vi "AuMT8852B Carrier Drift Test Configuration.vi"(5 "Settings":T1={"Low frequency selection"=enum."Use low frequency", "Medium frequency selection"=enum."Don't use medium frequency", "High frequency selection"=enum."Don't use high frequency", "Low TX frequency"=2402.0, "Medium TX frequency"=2441.0, "High TX frequency"=2480.0, "Number of packets"=10, "Hop selection"=enum."Test with hopping on", "DH1 selection"=enum."Test with DH1 packets", "DH3 selection"=enum."Test with DH3 packets", "DH5 selection"=enum."Test with DH5 packets", "1-slot packet drift limit"=25000.0, "3-slot packet drift limit"=40000.0, "5-slot packet drift limit"=40000.0, "Drift rate limit"=20000.0, "Test control"=enum."Loopback", "Hop mode"=enum."Defined", "Null packet drift limit"=20000.0, "Low RX frequency"=2480.0, "Medium RX frequency"=2402.0, "High RX frequency"=2402.0}, 7 "Set/Get (Set)":enum16{"Set", "Get"}(ring), 8 "error in (no error)":errorcluster, 10 "Script (3)":i32=3, 11 "VISA session":refnum<visa-resource-name>) -> (0 "error out":errorcluster, 2 "error code":i32, 3 "VISA session out":refnum<visa-resource-name>, 4 "Settings out":T1={"Low frequency selection"=enum."Use low frequency", "Medium frequency selection"=enum."Use medium frequency", "High frequency selection"=enum."Use high frequency", "Low TX frequency"=0.0, "Medium TX frequency"=0.0, "High TX frequency"=0.0, "Number of packets"=0, "Hop selection"=enum."Test with hopping on", "DH1 selection"=enum."Test with DH1 packets", "DH3 selection"=enum."Test with DH3 packets", "DH5 selection"=enum."Test with DH5 packets", "1-slot packet drift limit"=0.0, "3-slot packet drift limit"=0.0, "5-slot packet drift limit"=0.0, "Drift rate limit"=0.0, "Test control"=enum."Loopback", "Hop mode"=enum."Any", "Null packet drift limit"=0.0, "Low RX frequency"=0.0, "Medium RX frequency"=0.0, "High RX frequency"=0.0})   [LabVIEW 2017]
doc: "Anritsu MT8852B Bluetooth Tester\n\nConfigures the instrument for the Carrier Drift test.\n\nINPUTS\nSet/Get - whether the values are being sent to or retrieved from the instrument.\nScript - which of the stored scripts (1-10) will be queried or configured. Scripts 1 and 2 are read-only.\nSettings - parameters of the test to be written.\n\nOUTPUTS\nSettings out - current parameters of the test."
uses:
  <instrlib>/aumt8852B/General/Utilities/MT8850 Test Parameters.ctl
  <instrlib>/aumt8852B/General/Utilities/MT8850 Frequency Units.ctl
panel:
  in  "Case Constant\n(See Context Help)":bool
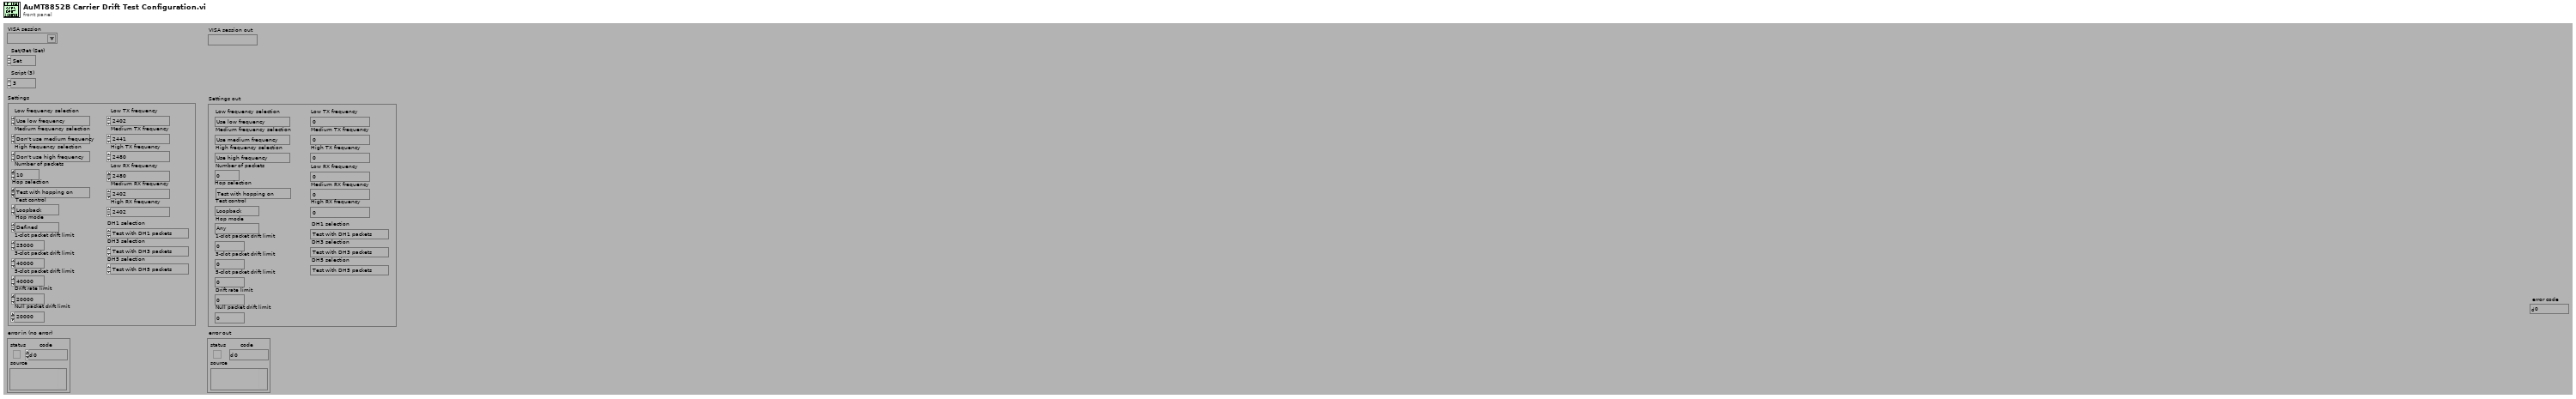
[diagram p1: front panel]
types:
  T1 = cluster{"Low frequency selection":enum16{"Don't use low frequency", "Use low frequency"}, "Medium frequency selection":enum16{"Don't use medium frequency", "Use medium frequency"}, "High frequency selection":enum16{"Don't use high frequency", "Use high frequency"}, "Low TX frequency":dbl, "Medium TX frequency":dbl, "High TX frequency":dbl, "Number of packets":i32, "Hop selection":enum16{"Test with hopping on", "Test with hopping off", "Test with hopping on and off"}, "DH1 selection":enum16{"Don't test with DH1 packets", "Test with DH1 packets"}, "DH3 selection":enum16{"Don't test with DH3 packets", "Test with DH3 packets"}, "DH5 selection":enum16{"Don't test with DH5 packets", "Test with DH5 packets"}, "1-slot packet drift limit":dbl, "3-slot packet drift limit":dbl, "5-slot packet drift limit":dbl, "Drift rate limit":dbl, "Test control":enum16{"Loopback", "TX test"}, "Hop mode":enum16{"All", "Any", "Defined"}, "Null packet drift limit":dbl, "Low RX frequency":dbl, "Medium RX frequency":dbl, "High RX frequency":dbl}
  T2 = typedef "MT8850 Test Parameters.ctl" = enum16{"Use low frequency", "Use medium frequency", "Use high frequency", "Low TX frequency", "Low RX frquency", "Medium TX frequency", "Medium RX frequency", "High TX frequency", "High RX frequency", "Number of packets", "Average high limit", "Average low limit", "Peak power limit", "Max power step limit", "Min power step limit", "f1 average minimum", "f1 average maximum", "f2 maximum", "f1/f2 average maximum", "Hop selection", "Use DH1 packets", "Use DH3 packets", "Use DH5 packets", "1 slot packet drift limit", "3 slot packet drift limit", "5 slot packet drift limit", "Drift rate limit", "TX power level", "Frequency offset", "Symbol timing", "Modulation index", "BER limit", "FER limit", "Use averaging high limit", "Use averaging low limit", "Use peak power limit", "Packet type", "Test control", "Use max power step limit", "Use min power step limit", "Number of cycles", "Use f1 average maximum", "Use f1 average minimum", "Use f2 maximum", "Use f1/f2 average maximum", "Hop mode", "Maximum negative limit", "Maximum positive limit", "Use maximum negative limit", "Use maximum positive limit", "Use 1 slot packet drift limit", "Use 3 slot packet drift limit", "Use 5 slot packet drift limit", "Use drift rate limit", "Use BER limit", "Use FER limit", "Use dirty parameter table", "Use null packet drift limit", "Null packet drift limit", "Minimum power", "Power delay", "Packet count", "Payload toggle", "Output power level", "2DHX packet type", "3DHX packet type", "Number of blocks", "TX and RX low frequency", "TX and RX medium frequency", "TX and RX high frequency", "TX frequency", "RX frequency", "Threshold bit count", "Total test bit count", "Number of bits", "PDPSK to PGFSK lower limit", "PDPSK to PGFSK upper limit", "Initial frequency error upper limit", "Initial frequency error lower limit", "Frequency error upper limit", "Frequency error lower limit", "Block frequency error upper limit", "Block frequency error lower limit", "2Mbs RMS DEVM limit", "3Mbs RMS DEVM limit", "2Mbs Peak DEVM limit", "3Mbs Peak DEVM limit", "2Mbs 99% packets DEVM limit", "3Mbs 99% packets DEVM limit", "Percentage of no error packets limit", "Threshold error limit", "Total test error limit"}
  T3 = typedef "MT8850 Frequency Units.ctl" = enum16{"Channel", "Hz", "kHz", "MHz", "GHz"}
  T4 = enum16{"Simulate", "Range check", "Cache", "Query instrument status"}
  T5 = enum16{"Output power", "Power control", "Modulation characteristics", "Initial carrier", "Carrier drift", "Single slot sensitivity", "Multiple slot sensitivity", "Maximum input power"}
  T6 = enum16{"Don't test with DH5 packets", "Test with DH5 packets"}
  T7 = enum16{"Don't test with DH3 packets", "Test with DH3 packets"}
  T8 = enum16{"Don't test with DH1 packets", "Test with DH1 packets"}
  T9 = enum16{"Test with hopping on", "Test with hopping off", "Test with hopping on and off"}
  T10 = enum16{"Don't use high frequency", "Use high frequency"}
  T11 = enum16{"Don't use medium frequency", "Use medium frequency"}
  T12 = enum16{"Don't use low frequency", "Use low frequency"}
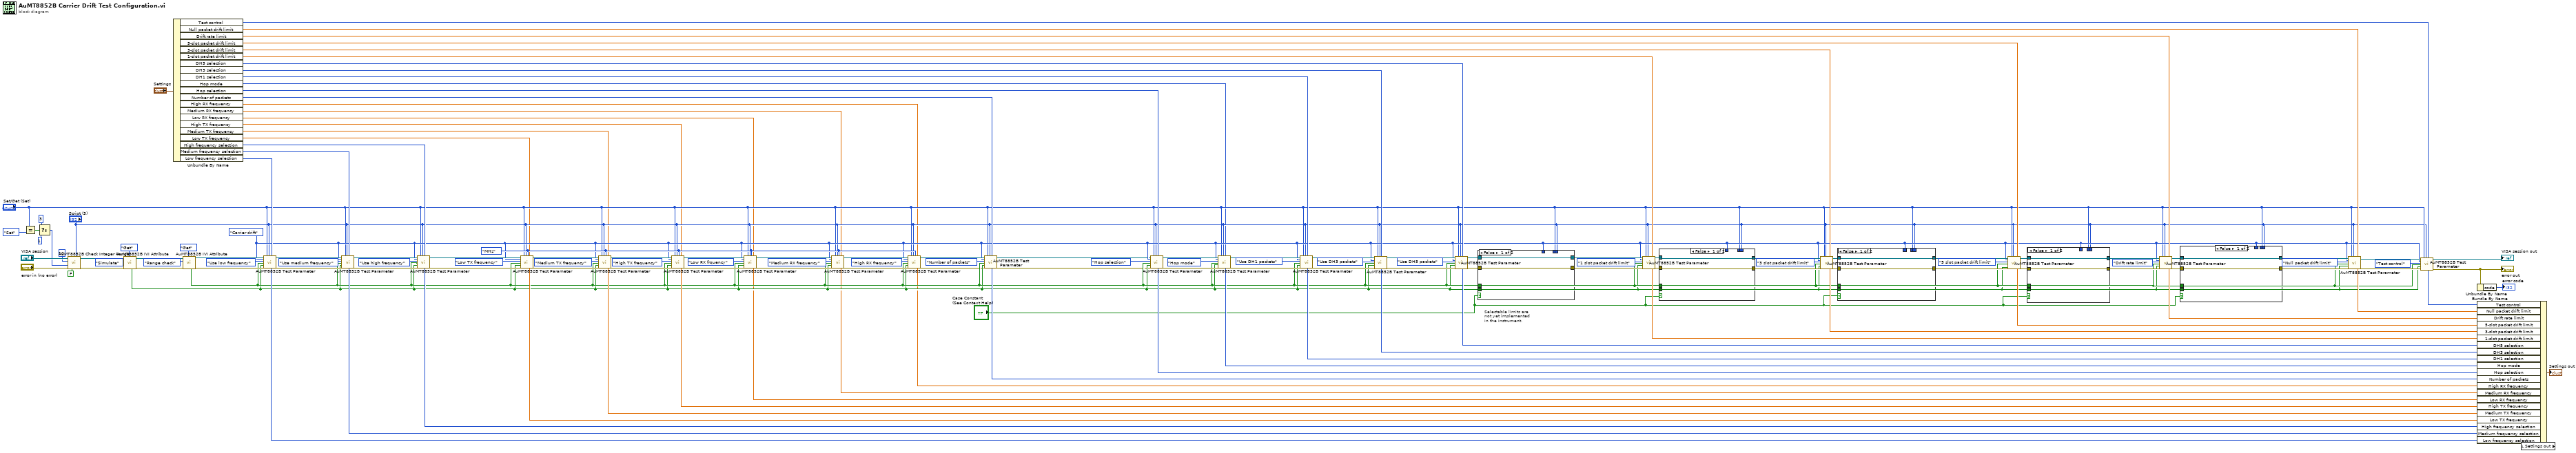
[diagram p0: block diagram]
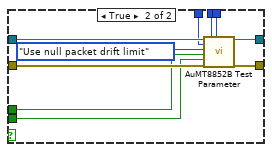
[diagram p2: hidden frame]
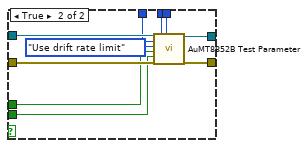
[diagram p3: hidden frame]
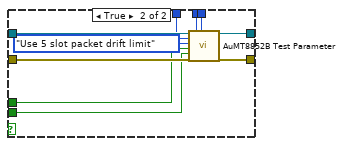
[diagram p4: hidden frame]
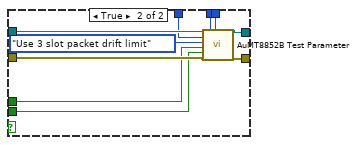
[diagram p5: hidden frame]
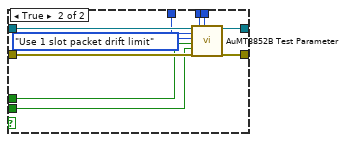
[diagram p6: hidden frame]
diagram:
  w20 = MT8850_Frequency_Units."MHz" ("Frequency units (MHz)")
  w15 = T5."Carrier drift" ("Test (Output Power)")
  # "Selectable limits are\nnot yet implemented\nin the instrument."
  n1 = Equal?(x="Set/Get (Set)", y=enum16{"Set", "Get"}."Set") -> (x = y?=w142:bool)
  n2 = Select(t=3, s=w142, f=1) -> (s? t:f=w138:i32)
  n3 = call <instrlib>:"AuMT8852B Check Integer Range.vi"("Value (0)"="Script (3)", "Check IVI flag first? (T)"=FALSE, "error in (no error)"="error in (no error)", "Lower limit (-1)"=w138, "Upper limit (1)"=10, "VISA session"="VISA session") -> ("error out"=w136:errorcluster, "VISA session out"=w137:refnum<visa-resource-name>)  [unwired: 4 in]
  n4 = call <instrlib>:"AuMT8852B IVI Attribute.vi"("Set/Get (Set)"=enum16{"Set", "Get"}."Get", "error in (no error)"=w136, "Flag (Simulate)"=T4."Simulate", "VISA session"=w137) -> ("error out"=w117:errorcluster, "VISA session out"=w118:refnum<visa-resource-name>, "Value out"=w18:bool)  [unwired: 5 in]
  n5 = Unbundle By Name("Settings") -> ("Test control"=w33:enum16{"Loopback", "TX test"}, "Null packet drift limit"=w34:dbl, "Drift rate limit"=w83:dbl, "5-slot packet drift limit"=w84:dbl, "3-slot packet drift limit"=w85:dbl, "1-slot packet drift limit"=w86:dbl, "DH5 selection"=w87:T6, "DH3 selection"=w88:T7, "DH1 selection"=w89:T8, "Hop mode"=w1:enum16{"All", "Any", "Defined"}, "Hop selection"=w96:T9, "Number of packets"=w108:i32, "High RX frequency"=w9:dbl, "Medium RX frequency"=w8:dbl, "Low RX frequency"=w2:dbl, "High TX frequency"=w10:dbl, "Medium TX frequency"=w11:dbl, "Low TX frequency"=w12:dbl, "High frequency selection"=w109:T10, "Medium frequency selection"=w110:T11, "Low frequency selection"=w111:T12)
  n6 = call <instrlib>:"AuMT8852B IVI Attribute.vi"("Set/Get (Set)"=enum16{"Set", "Get"}."Get", "error in (no error)"=w117, "Flag (Simulate)"=T4."Range check", "VISA session"=w118) -> ("error out"=w115:errorcluster, "VISA session out"=w116:refnum<visa-resource-name>, "Value out"=w19:bool)  [unwired: 5 in]
  n7 = call <instrlib>:"AuMT8852B Test Parameter.vi"("VISA session"=w116, "Test (Output power)"=w15, "Parameter (Use low frequency)"=MT8850_Test_Parameters."Use low frequency", "Range check? (F)"=w19, "Simulate? (F)"=w18, "error in (no error)"=w115, "Set/Get (Set)"="Set/Get (Set)", "Script (3)"="Script (3)", "Integer value (0)"=w111) -> ("Integer value out"=w100:i32, "VISA session out"=w49:refnum<visa-resource-name>, "error out"=w48:errorcluster)  [unwired: 7 in, 1 out]
  n8 = call <instrlib>:"AuMT8852B Test Parameter.vi"("VISA session"=w49, "Test (Output power)"=w15, "Parameter (Use low frequency)"=MT8850_Test_Parameters."Use medium frequency", "Range check? (F)"=w19, "Simulate? (F)"=w18, "error in (no error)"=w48, "Set/Get (Set)"="Set/Get (Set)", "Script (3)"="Script (3)", "Integer value (0)"=w110) -> ("Integer value out"=w101:i32, "VISA session out"=w47:refnum<visa-resource-name>, "error out"=w46:errorcluster)  [unwired: 7 in, 1 out]
  n9 = call <instrlib>:"AuMT8852B Test Parameter.vi"("VISA session"=w47, "Test (Output power)"=w15, "Parameter (Use low frequency)"=MT8850_Test_Parameters."Use high frequency", "Range check? (F)"=w19, "Simulate? (F)"=w18, "error in (no error)"=w46, "Set/Get (Set)"="Set/Get (Set)", "Script (3)"="Script (3)", "Integer value (0)"=w109) -> ("Integer value out"=w102:i32, "VISA session out"=w132:refnum<visa-resource-name>, "error out"=w131:errorcluster)  [unwired: 7 in, 1 out]
  n10 = call <instrlib>:"AuMT8852B Test Parameter.vi"("VISA session"=w132, "Test (Output power)"=w15, "Parameter (Use low frequency)"=MT8850_Test_Parameters."Low TX frequency", "Range check? (F)"=w19, "Simulate? (F)"=w18, "error in (no error)"=w131, "Set/Get (Set)"="Set/Get (Set)", "Script (3)"="Script (3)", "Integer value (0)"=w20, "Float value (0)"=w12) -> ("Float value out"=w103:dbl, "VISA session out"=w130:refnum<visa-resource-name>, "error out"=w129:errorcluster)  [unwired: 6 in, 1 out]
  n11 = call <instrlib>:"AuMT8852B Test Parameter.vi"("VISA session"=w130, "Test (Output power)"=w15, "Parameter (Use low frequency)"=MT8850_Test_Parameters."Medium TX frequency", "Range check? (F)"=w19, "Simulate? (F)"=w18, "error in (no error)"=w129, "Set/Get (Set)"="Set/Get (Set)", "Script (3)"="Script (3)", "Integer value (0)"=w20, "Float value (0)"=w11) -> ("Float value out"=w104:dbl, "VISA session out"=w128:refnum<visa-resource-name>, "error out"=w127:errorcluster)  [unwired: 6 in, 1 out]
  n12 = call <instrlib>:"AuMT8852B Test Parameter.vi"("VISA session"=w128, "Test (Output power)"=w15, "Parameter (Use low frequency)"=MT8850_Test_Parameters."High TX frequency", "Range check? (F)"=w19, "Simulate? (F)"=w18, "error in (no error)"=w127, "Set/Get (Set)"="Set/Get (Set)", "Script (3)"="Script (3)", "Integer value (0)"=w20, "Float value (0)"=w10) -> ("Float value out"=w105:dbl, "VISA session out"=w22:refnum<visa-resource-name>, "error out"=w21:errorcluster)  [unwired: 6 in, 1 out]
  n13 = call <instrlib>:"AuMT8852B Test Parameter.vi"("VISA session"=w22, "Test (Output power)"=w15, "Parameter (Use low frequency)"=MT8850_Test_Parameters."Low RX frquency", "Range check? (F)"=w19, "Simulate? (F)"=w18, "error in (no error)"=w21, "Set/Get (Set)"="Set/Get (Set)", "Script (3)"="Script (3)", "Integer value (0)"=w20, "Float value (0)"=w2) -> ("Float value out"=w5:dbl, "VISA session out"=w23:refnum<visa-resource-name>, "error out"=w24:errorcluster)  [unwired: 6 in, 1 out]
  n14 = call <instrlib>:"AuMT8852B Test Parameter.vi"("VISA session"=w23, "Test (Output power)"=w15, "Parameter (Use low frequency)"=MT8850_Test_Parameters."Medium RX frequency", "Range check? (F)"=w19, "Simulate? (F)"=w18, "error in (no error)"=w24, "Set/Get (Set)"="Set/Get (Set)", "Script (3)"="Script (3)", "Integer value (0)"=w20, "Float value (0)"=w8) -> ("Float value out"=w6:dbl, "VISA session out"=w25:refnum<visa-resource-name>, "error out"=w26:errorcluster)  [unwired: 6 in, 1 out]
  n15 = call <instrlib>:"AuMT8852B Test Parameter.vi"("VISA session"=w25, "Test (Output power)"=w15, "Parameter (Use low frequency)"=MT8850_Test_Parameters."High RX frequency", "Range check? (F)"=w19, "Simulate? (F)"=w18, "error in (no error)"=w26, "Set/Get (Set)"="Set/Get (Set)", "Script (3)"="Script (3)", "Integer value (0)"=w20, "Float value (0)"=w9) -> ("Float value out"=w7:dbl, "VISA session out"=w16:refnum<visa-resource-name>, "error out"=w17:errorcluster)  [unwired: 6 in, 1 out]
  n16 = call <instrlib>:"AuMT8852B Test Parameter.vi"("VISA session"=w16, "Test (Output power)"=w15, "Parameter (Use low frequency)"=MT8850_Test_Parameters."Number of packets", "Range check? (F)"=w19, "Simulate? (F)"=w18, "error in (no error)"=w17, "Set/Get (Set)"="Set/Get (Set)", "Script (3)"="Script (3)", "Integer value (0)"=w108) -> ("Integer value out"=w106:i32, "VISA session out"=w4:refnum<visa-resource-name>, "error out"=w3:errorcluster)  [unwired: 7 in, 1 out]
  n17 = call <instrlib>:"AuMT8852B Test Parameter.vi"("VISA session"=w4, "Test (Output power)"=w15, "Parameter (Use low frequency)"=MT8850_Test_Parameters."Hop selection", "Range check? (F)"=w19, "Simulate? (F)"=w18, "error in (no error)"=w3, "Set/Get (Set)"="Set/Get (Set)", "Script (3)"="Script (3)", "Integer value (0)"=w96) -> ("Integer value out"=w95:i32, "VISA session out"=w126:refnum<visa-resource-name>, "error out"=w125:errorcluster)  [unwired: 7 in, 1 out]
  n18 = call <instrlib>:"AuMT8852B Test Parameter.vi"("VISA session"=w126, "Test (Output power)"=w15, "Parameter (Use low frequency)"=MT8850_Test_Parameters."Hop mode", "Range check? (F)"=w19, "Simulate? (F)"=w18, "error in (no error)"=w125, "Set/Get (Set)"="Set/Get (Set)", "Script (3)"="Script (3)", "Integer value (0)"=w1) -> ("Integer value out"=w94:i32, "VISA session out"=w99:refnum<visa-resource-name>, "error out"=w98:errorcluster)  [unwired: 7 in, 1 out]
  n19 = call <instrlib>:"AuMT8852B Test Parameter.vi"("VISA session"=w99, "Test (Output power)"=w15, "Parameter (Use low frequency)"=MT8850_Test_Parameters."Use DH1 packets", "Range check? (F)"=w19, "Simulate? (F)"=w18, "error in (no error)"=w98, "Set/Get (Set)"="Set/Get (Set)", "Script (3)"="Script (3)", "Integer value (0)"=w89) -> ("Integer value out"=w70:i32, "VISA session out"=w93:refnum<visa-resource-name>, "error out"=w92:errorcluster)  [unwired: 7 in, 1 out]
  n20 = call <instrlib>:"AuMT8852B Test Parameter.vi"("VISA session"=w93, "Test (Output power)"=w15, "Parameter (Use low frequency)"=MT8850_Test_Parameters."Use DH3 packets", "Range check? (F)"=w19, "Simulate? (F)"=w18, "error in (no error)"=w92, "Set/Get (Set)"="Set/Get (Set)", "Script (3)"="Script (3)", "Integer value (0)"=w88) -> ("Integer value out"=w71:i32, "VISA session out"=w91:refnum<visa-resource-name>, "error out"=w90:errorcluster)  [unwired: 7 in, 1 out]
  n21 = call <instrlib>:"AuMT8852B Test Parameter.vi"("VISA session"=w91, "Test (Output power)"=w15, "Parameter (Use low frequency)"=MT8850_Test_Parameters."Use DH5 packets", "Range check? (F)"=w19, "Simulate? (F)"=w18, "error in (no error)"=w90, "Set/Get (Set)"="Set/Get (Set)", "Script (3)"="Script (3)", "Integer value (0)"=w87) -> ("Integer value out"=w72:i32, "VISA session out"=w56:refnum<visa-resource-name>, "error out"=w57:errorcluster)  [unwired: 7 in, 1 out]
  n22 = case shown="False" "Case Constant\n(See Context Help)" {
    tunnel: w57 -> [w146 w156]
    tunnel: w56 -> [w147 w155]
    tunnel: [w147 w154] -> w55
    tunnel: [w146 w153] -> w54
    tunnel: w15 -> [_ w152]
    tunnel: "Set/Get (Set)" -> [_ w151]
    tunnel: "Script (3)" -> [_ w150]
    tunnel: w18 -> [_ w149]
    tunnel: w19 -> [_ w148]
    frame False {
    }
    frame True {
      n23 = call <instrlib>:"AuMT8852B Test Parameter.vi"("VISA session"=w155, "Test (Output power)"=w152, "Parameter (Use low frequency)"=MT8850_Test_Parameters."Use 1 slot packet drift limit", "Range check? (F)"=w148, "Simulate? (F)"=w149, "error in (no error)"=w156, "Set/Get (Set)"=w151, "Script (3)"=w150) -> ("VISA session out"=w154:refnum<visa-resource-name>, "error out"=w153:errorcluster)  [unwired: 8 in, 2 out]
    }
  }
  n24 = call <instrlib>:"AuMT8852B Test Parameter.vi"("VISA session"=w55, "Test (Output power)"=w15, "Parameter (Use low frequency)"=MT8850_Test_Parameters."1 slot packet drift limit", "Range check? (F)"=w19, "Simulate? (F)"=w18, "error in (no error)"=w54, "Set/Get (Set)"="Set/Get (Set)", "Script (3)"="Script (3)", "Float value (0)"=w86) -> ("Float value out"=w73:dbl, "VISA session out"=w58:refnum<visa-resource-name>, "error out"=w61:errorcluster)  [unwired: 7 in, 1 out]
  n25 = case shown="False" "Case Constant\n(See Context Help)" {
    tunnel: w61 -> [w159 w168]
    tunnel: [w159 w167] -> w60
    tunnel: [w158 w166] -> w59
    tunnel: w58 -> [w158 w165]
    tunnel: w15 -> [_ w164]
    tunnel: "Set/Get (Set)" -> [_ w163]
    tunnel: "Script (3)" -> [_ w162]
    tunnel: w18 -> [_ w161]
    tunnel: w19 -> [_ w160]
    frame False {
    }
    frame True {
      n26 = call <instrlib>:"AuMT8852B Test Parameter.vi"("VISA session"=w165, "Test (Output power)"=w164, "Parameter (Use low frequency)"=MT8850_Test_Parameters."Use 3 slot packet drift limit", "Range check? (F)"=w160, "Simulate? (F)"=w161, "error in (no error)"=w168, "Set/Get (Set)"=w163, "Script (3)"=w162) -> ("VISA session out"=w166:refnum<visa-resource-name>, "error out"=w167:errorcluster)  [unwired: 8 in, 2 out]
    }
  }
  n27 = call <instrlib>:"AuMT8852B Test Parameter.vi"("VISA session"=w59, "Test (Output power)"=w15, "Parameter (Use low frequency)"=MT8850_Test_Parameters."3 slot packet drift limit", "Range check? (F)"=w19, "Simulate? (F)"=w18, "error in (no error)"=w60, "Set/Get (Set)"="Set/Get (Set)", "Script (3)"="Script (3)", "Float value (0)"=w85) -> ("Float value out"=w74:dbl, "VISA session out"=w62:refnum<visa-resource-name>, "error out"=w65:errorcluster)  [unwired: 7 in, 1 out]
  n28 = case shown="False" "Case Constant\n(See Context Help)" {
    tunnel: w65 -> [w170 w180]
    tunnel: [w170 w179] -> w64
    tunnel: [w171 w178] -> w63
    tunnel: w62 -> [w171 w177]
    tunnel: w15 -> [_ w176]
    tunnel: "Set/Get (Set)" -> [_ w175]
    tunnel: "Script (3)" -> [_ w174]
    tunnel: w18 -> [_ w173]
    tunnel: w19 -> [_ w172]
    frame False {
    }
    frame True {
      n29 = call <instrlib>:"AuMT8852B Test Parameter.vi"("VISA session"=w177, "Test (Output power)"=w176, "Parameter (Use low frequency)"=MT8850_Test_Parameters."Use 5 slot packet drift limit", "Range check? (F)"=w172, "Simulate? (F)"=w173, "error in (no error)"=w180, "Set/Get (Set)"=w175, "Script (3)"=w174) -> ("VISA session out"=w178:refnum<visa-resource-name>, "error out"=w179:errorcluster)  [unwired: 8 in, 2 out]
    }
  }
  n30 = call <instrlib>:"AuMT8852B Test Parameter.vi"("VISA session"=w63, "Test (Output power)"=w15, "Parameter (Use low frequency)"=MT8850_Test_Parameters."5 slot packet drift limit", "Range check? (F)"=w19, "Simulate? (F)"=w18, "error in (no error)"=w64, "Set/Get (Set)"="Set/Get (Set)", "Script (3)"="Script (3)", "Float value (0)"=w84) -> ("Float value out"=w75:dbl, "VISA session out"=w69:refnum<visa-resource-name>, "error out"=w68:errorcluster)  [unwired: 7 in, 1 out]
  n31 = case shown="False" "Case Constant\n(See Context Help)" {
    tunnel: w69 -> [w182 w192]
    tunnel: w68 -> [w183 w191]
    tunnel: [w183 w190] -> w67
    tunnel: [w182 w189] -> w66
    tunnel: w15 -> [_ w188]
    tunnel: w18 -> [_ w187]
    tunnel: w19 -> [_ w186]
    tunnel: "Set/Get (Set)" -> [_ w185]
    tunnel: "Script (3)" -> [_ w184]
    frame False {
    }
    frame True {
      n32 = call <instrlib>:"AuMT8852B Test Parameter.vi"("VISA session"=w192, "Test (Output power)"=w188, "Parameter (Use low frequency)"=MT8850_Test_Parameters."Use drift rate limit", "Range check? (F)"=w186, "Simulate? (F)"=w187, "error in (no error)"=w191, "Set/Get (Set)"=w185, "Script (3)"=w184) -> ("VISA session out"=w189:refnum<visa-resource-name>, "error out"=w190:errorcluster)  [unwired: 8 in, 2 out]
    }
  }
  n33 = call <instrlib>:"AuMT8852B Test Parameter.vi"("VISA session"=w66, "Test (Output power)"=w15, "Parameter (Use low frequency)"=MT8850_Test_Parameters."Drift rate limit", "Range check? (F)"=w19, "Simulate? (F)"=w18, "error in (no error)"=w67, "Set/Get (Set)"="Set/Get (Set)", "Script (3)"="Script (3)", "Float value (0)"=w83) -> ("Float value out"=w76:dbl, "VISA session out"=w41:refnum<visa-resource-name>, "error out"=w40:errorcluster)  [unwired: 7 in, 1 out]
  n34 = case shown="False" "Case Constant\n(See Context Help)" {
    tunnel: w41 -> [w194 w204]
    tunnel: w40 -> [w195 w203]
    tunnel: [w195 w202] -> w38
    tunnel: [w194 w201] -> w37
    tunnel: w15 -> [_ w200]
    tunnel: "Set/Get (Set)" -> [_ w199]
    tunnel: "Script (3)" -> [_ w198]
    tunnel: w19 -> [_ w197]
    tunnel: w18 -> [_ w196]
    frame False {
    }
    frame True {
      n35 = call <instrlib>:"AuMT8852B Test Parameter.vi"("VISA session"=w204, "Test (Output power)"=w200, "Parameter (Use low frequency)"=MT8850_Test_Parameters."Use null packet drift limit", "Range check? (F)"=w197, "Simulate? (F)"=w196, "error in (no error)"=w203, "Set/Get (Set)"=w199, "Script (3)"=w198) -> ("VISA session out"=w201:refnum<visa-resource-name>, "error out"=w202:errorcluster)  [unwired: 8 in, 2 out]
    }
  }
  n36 = call <instrlib>:"AuMT8852B Test Parameter.vi"("VISA session"=w37, "Test (Output power)"=w15, "Parameter (Use low frequency)"=MT8850_Test_Parameters."Null packet drift limit", "Range check? (F)"=w19, "Simulate? (F)"=w18, "error in (no error)"=w38, "Set/Get (Set)"="Set/Get (Set)", "Script (3)"="Script (3)", "Float value (0)"=w34) -> ("Float value out"=w31:dbl, "VISA session out"=w35:refnum<visa-resource-name>, "error out"=w36:errorcluster)  [unwired: 7 in, 1 out]
  n37 = call <instrlib>:"AuMT8852B Test Parameter.vi"("VISA session"=w35, "Test (Output power)"=w15, "Parameter (Use low frequency)"=MT8850_Test_Parameters."Test control", "Range check? (F)"=w19, "Simulate? (F)"=w18, "error in (no error)"=w36, "Set/Get (Set)"="Set/Get (Set)", "Script (3)"="Script (3)", "Integer value (0)"=w33) -> ("Integer value out"=w32:i32, "VISA session out"=→"VISA session out":refnum<visa-resource-name>, "error out"=w42:errorcluster)  [unwired: 7 in, 1 out]
  "error out" <- w42
  n38 = Unbundle By Name(w42) -> ("code"=→"error code":i32)
  n39 = local read "Settings out"() -> (w107:T1)
  n40 = Bundle By Name(cluster=w107, "Test control"=w32, "Null packet drift limit"=w31, "Drift rate limit"=w76, "5-slot packet drift limit"=w75, "3-slot packet drift limit"=w74, "1-slot packet drift limit"=w73, "DH5 selection"=w72, "DH3 selection"=w71, "DH1 selection"=w70, "Hop mode"=w94, "Hop selection"=w95, "Number of packets"=w106, "High RX frequency"=w7, "Medium RX frequency"=w6, "Low RX frequency"=w5, "High TX frequency"=w105, "Medium TX frequency"=w104, "Low TX frequency"=w103, "High frequency selection"=w102, "Medium frequency selection"=w101, "Low frequency selection"=w100) -> (→"Settings out":T1)
